vi "Max AI (SubVI).vi"(8 "Threshold":i16, 9 "AI Scan Period (us)":u32, 10 "Digital Output":refnum<k21>="Connector0/DIO0", 11 "Analog Input":refnum<k21>="Connector0/AI0") -> (1 "Threshold Reached":bool, 2 "AI value":i16)   [LabVIEW 2012]
doc: "This VI monitors a user-selectable analog input channel and controls a user-selectable digital output line after waiting a set amount of time."
uses:
  <vilib>/rvi/eio/common/nirviEmuTemplateMethod_errors.vi
  <vilib>/eio/EIONode/EIONode.xnode
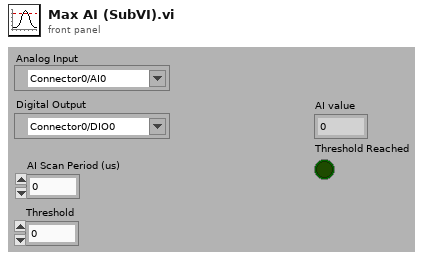
[diagram p1: front panel]
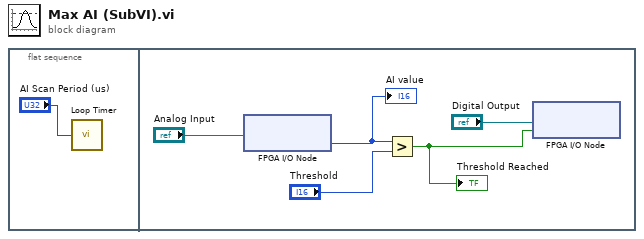
[diagram p0: block diagram]
diagram:
  n1 = flat-sequence {
    frame #0 {
      n2 = call "Loop Timer"("Count(uSec)"="AI Scan Period (us)") -> ()  [unwired: 1 out]
    }
    frame #1 {
      n3 = xnode "FPGA I/O Node"("FPGA I/O In"="Analog Input") -> ("I/O Item"=w5:i16)  [unwired: 1 out]
      "AI value" <- w5
      n4 = Greater?(x=w5, y="Threshold") -> (0:w2:bool)
      "Threshold Reached" <- w2
      n5 = xnode "FPGA I/O Node"("I/O Item"=w2, "FPGA I/O In"="Digital Output") -> ()  [unwired: 1 out]
    }
  }
